vi "RobotState_get.vi"(8 "error in (no error)":errorcluster) -> (0 "error out":errorcluster, 2 "RobotState":T1)   [LabVIEW 2009, in "NetworkVarTarget.lvlib"]
uses:
  NetworkVarTarget.lvlib
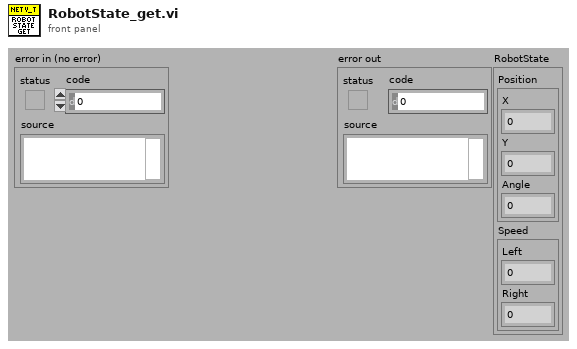
[diagram p1: front panel]
types:
  T1 = cluster{"Position":cluster{"X":dbl, "Y":dbl, "Angle":dbl}, "Speed":cluster{"Left":dbl, "Right":dbl}}
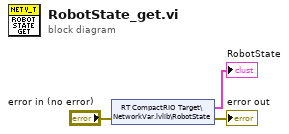
[diagram p0: block diagram]
diagram:
  n1 = shared-variable "RT CompactRIO Target\\NetworkVar.lvlib\\RobotState"(error in="error in (no error)") -> (→"RobotState":T1, error out=→"error out":errorcluster)
